vi "rs3 get frame width.vi"(8 "error in (no error)":errorcluster, 11 "frame in":u64) -> (0 "error out":errorcluster, 1 "error":u64, 2 "width":i32, 3 "Frame out":u64)   [LabVIEW 2017, in "libRealSense3.lvlib"]
doc: "Returns the FRAME width."
uses:
  <vilib>/addons/RealSense/libRealSense3.lvlib
  Users/Greg McKaskle/Downloads/librealsense-1.12.1/librealsense-1.12.1/bin/Win32/realsense-d.dll
panel:
  # "RS3 Get Frame Width"
  # "(C) Intel Corp. 2017,  AGJ"
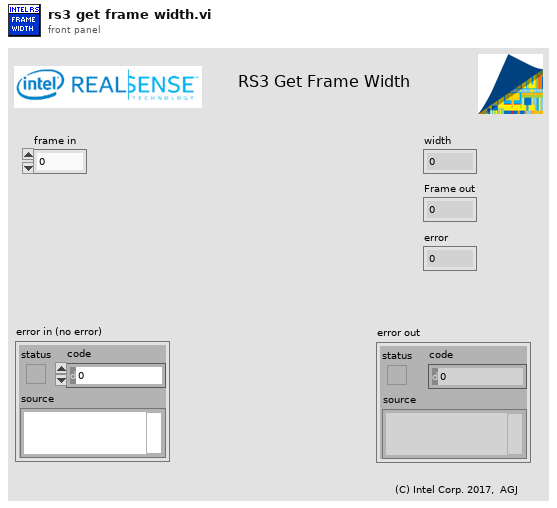
[diagram p1: front panel]
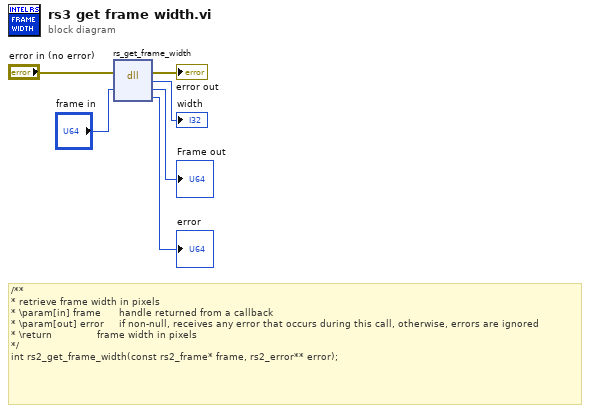
[diagram p0: block diagram]
diagram:
  # "/**\n* retrieve frame width in pixels\n* \\param[in] frame      handle returned from a callback\n* \\param[out] error     if non-null, receives any error that occurs during this call, otherwise, errors are ignored\n* \\return               frame width in pixels\n*/\nint rs2_get_frame_width(const rs2_frame* frame, rs2_error** error);"
  n1 = dll-call lib="C:/Users/Greg McKaskle/Downloads/librealsense-1.12.1/librealsense-1.12.1/bin/Win32/realsense-d.dll" fn="rs_get_frame_width"(error in="error in (no error)", "frame"="frame in") -> (error out=→"error out":errorcluster, "width"=→"width":i32, "frame"=→"Frame out":u64, "error"=→"error":u64)  [unwired: 3 in, 1 out]
